vi "Expand Special Cluster.vi"(6 "Special Terminal Indices in":T5={"Action"=-1, "Init"=-1, "Tag"=-1, "State in"=-1, "State out"=-1, "Error"=-1}, 9 "Type Descriptor":T2, 10 "Special Terminal":T1, 11 "Variant":variant) -> (0 "Save Types?":bool, 1 "Contained Types":T2[](array[typedef]), 4 "Special Terminal Indices":T5={"Action"=-1, "Init"=-1, "Tag"=-1, "State in"=-1, "State out"=-1, "Error"=-1})   [LabVIEW 2022 SP3, in "FlexBlocks Support.lvlib"]
uses:
  FlexBlocks Support.lvlib
  <vilib>/Utility/Data Type/NI_Data Type.lvlib
  Special Terminal Indices.ctl
  Terminal Direction.ctl
  Value Mode.ctl
  Special Terminal.ctl
  Type Descriptor.ctl
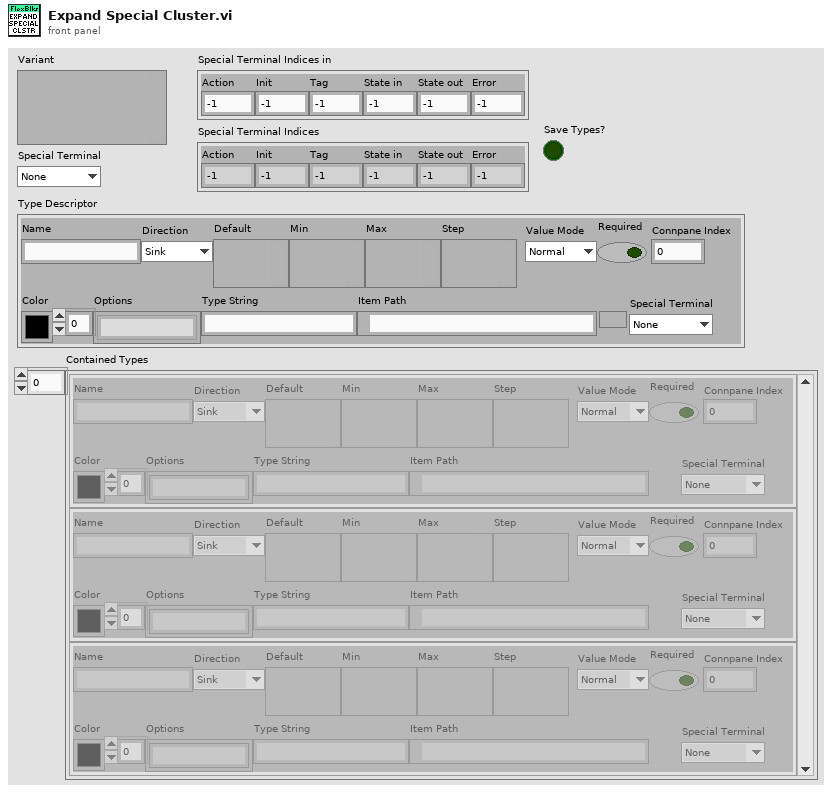
[diagram p1: front panel]
types:
  T1 = typedef "FlexBlocks Support.lvlib/Special Terminal.ctl" = enum16{"None", "Action", "Init", "Tag", "State in", "State out", "Error"}
  T2 = typedef "FlexBlocks Support.lvlib/Type Descriptor.ctl" = cluster{"Name":string, "Direction":T3, "Default":variant, "Min":variant, "Max":variant, "Step":variant, "Value Mode":T4, "Color":u32, "Options":string[], "Type String":string, "Item Path":path, "Required":bool, "Connpane Index":i32, "Special Terminal":T1}
  T3 = typedef "FlexBlocks Support.lvlib/Terminal Direction.ctl" = enum16{"Sink", "Source"}
  T4 = typedef "FlexBlocks Support.lvlib/Value Mode.ctl" = enum16{"Normal", "Range", "Select"}
  T5 = typedef "FlexBlocks Support.lvlib/Special Terminal Indices.ctl" = cluster{"Action":i32, "Init":i32, "Tag":i32, "State in":i32, "State out":i32, "Error":i32}
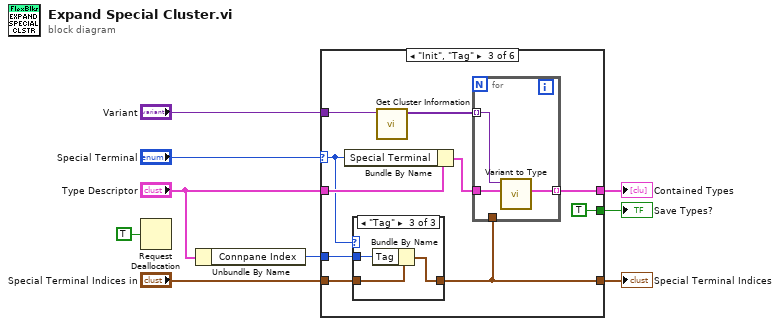
[diagram p0: block diagram]
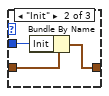
[diagram p5: hidden frame]
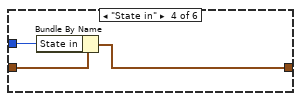
[diagram p6: hidden frame]
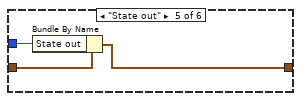
[diagram p7: hidden frame]
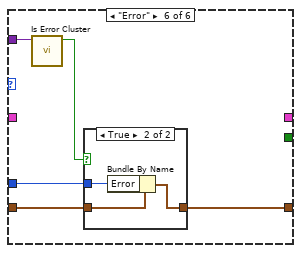
[diagram p8: hidden frame]
diagram:
  n1 = Request Deallocation(TRUE ("flag")) -> ()
  n2 = Unbundle By Name("Type Descriptor") -> ("Connpane Index"=w2:i32)
  n3 = case shown="\"Init\", \"Tag\"" "Special Terminal" {
    selector: "Special Terminal" -> [_ _ w16 _ _ _]
    tunnel: "Type Descriptor" -> [_ _ w20 _ _ _]
    tunnel: "Variant" -> [_ _ w21 _ _ w42]
    tunnel: "Special Terminal Indices in" -> [w10 w11 w14 w34 w37 w41]
    tunnel: [w10 w11 w13 w33 w36 w38] -> w4
    tunnel: [_ _ w19 _ _ _] -> w3
    tunnel: w2 -> [_ _ w15 w32 w35 w40]
    tunnel: [_ _ TRUE _ _ _] -> w1
    frame "None" {
    }
    frame "Action" {
    }
    frame "Init", "Tag" {
      n4 = Bundle By Name(cluster=w20, "Special Terminal"=w16) -> (w18:T2)
      n5 = case shown="\"Tag\"" w16 {
        tunnel: w15 -> [_ w24 w27]
        tunnel: w14 -> [w22 w25 w28]
        tunnel: [w22 w23 w26] -> w13
        frame Default {
        }
        frame "Init" {
          n6 = Bundle By Name(cluster=w25, "Init"=w24) -> (w23:T5)
        }
        frame "Tag" {
          n7 = Bundle By Name(cluster=w28, "Tag"=w27) -> (w26:T5)
        }
      }
      n8 = call <vilib>:"Get Cluster Information.vi"("variant"=w21) -> ("cluster elements"=w17:variant[])  [unwired: 9 in, 1 out]
      n9 = for {
        tunnel: w18 -> [w31]
        tunnel: [w30] -> w19 mode=indexing
        tunnel: w17 -> [w29] mode=indexing
        tunnel: w13 -> [_]
        n10 = call "Variant to Type.vi"("Type Descriptor in"=w31, "Variant"=w29) -> ("Type Descriptor"=w30:T2)  [unwired: 9 in]
      }
    }
    frame "State in" {
      n11 = Bundle By Name(cluster=w34, "State in"=w32) -> (w33:T5)
    }
    frame "State out" {
      n12 = Bundle By Name(cluster=w37, "State out"=w35) -> (w36:T5)
    }
    frame "Error" {
      n13 = call <vilib>:"Is Error Cluster.vi"("variant"=w42) -> ("is error cluster?"=w39:bool)  [unwired: 9 in, 1 out]
      n14 = case shown="True" w39 {
        tunnel: w41 -> [w43 w46]
        tunnel: w40 -> [_ w45]
        tunnel: [w43 w44] -> w38
        frame False {
        }
        frame True {
          n15 = Bundle By Name(cluster=w46, "Error"=w45) -> (w44:T5)
        }
      }
    }
  }
  "Special Terminal Indices" <- w4
  "Save Types?" <- w1
  "Contained Types" <- w3
